vi "Close-file.vi"(8 "error in (no error)":errorcluster, 11 "SettingsFile in":refnum<class "SettingsFile.lvclass">) -> (0 "error out":errorcluster, 3 "SettingsFile out":refnum<class "SettingsFile.lvclass">)   [LabVIEW 2013, in "SettingsFile.lvlib" / "SettingsFile.lvclass"]
uses:
  SettingsFile.lvclass
  SettingsFile.lvclass/SettingsFile.ctl
  Errors.ctl
  <vilib>/Utility/config.llb/Config Data RefNum.ctl
  <vilib>/Utility/config.llb/NI_LVConfig.lvlib
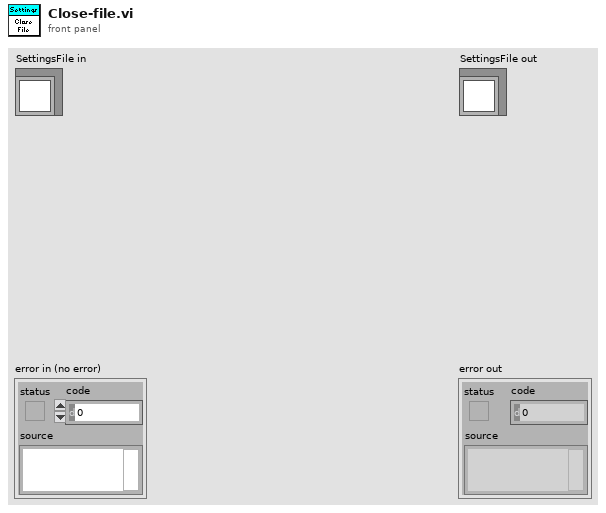
[diagram p1: front panel]
types:
  T1 = typedef "SettingsFile.lvlib/SettingsFile.lvclass/Errors.ctl" = enum16{"Not implemented", "Command not recognized", "Invalid input", "No connection", "Timeout", "Invalid file type", "No file access"}
  T2 = typedef "NI_LVConfig.lvlib/Config Data RefNum.ctl" = refnum<k1>
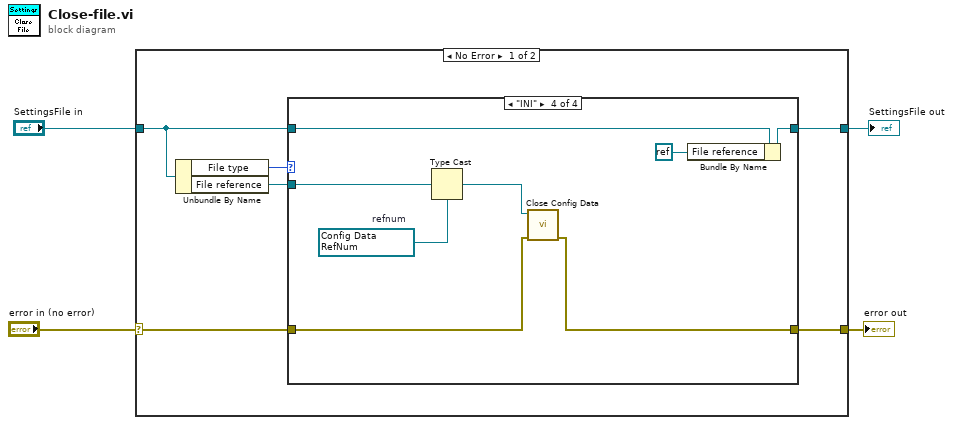
[diagram p0: block diagram]
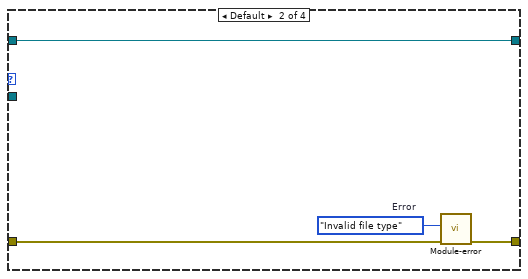
[diagram p3: hidden frame]
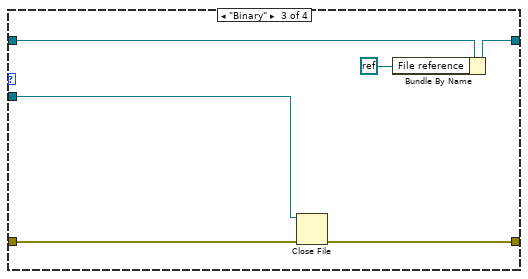
[diagram p4: hidden frame]
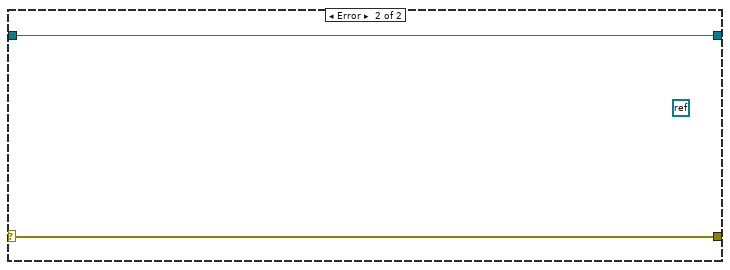
[diagram p5: hidden frame]
diagram:
  n1 = case shown="No Error" "error in (no error)" {
    selector: "error in (no error)" -> [w10 w32]
    tunnel: [w9 w32] -> w3
    tunnel: [w8 w31] -> w1
    tunnel: "SettingsFile in" -> [w7 w31]
    frame No Error {
      n2 = Unbundle By Name(w7) -> ("File type"=w6:enum16{"XML", "INI", "Binary"}, "File reference"=w5:refnum<file>)
      n3 = case shown="\"INI\"" w6 {
        tunnel: w7 -> [w12 w16 w22 w30]
        tunnel: w10 -> [w11 w14 w20 w27]
        tunnel: [w11 w15 w19 w26] -> w9
        tunnel: [w12 w16 w21 w29] -> w8
        tunnel: w5 -> [_ _ w18 w28]
        frame "XML" {
        }
        frame Default {
          w13 = Errors."Invalid file type"  # Error
          n4 = call "Module-error.vi"("error in (no error)"=w14, "Error"=w13) -> ("error out"=w15:errorcluster)  [unwired: 9 in]
        }
        frame "Binary" {
          n5 = Close File(refnum=w18, error in=w20) -> (error out=w19:errorcluster)  [unwired: 1 out]
          n6 = Bundle By Name(cluster=w22, "File reference"=refnum<k0> refnum) -> (w21:refnum<class "SettingsFile.lvclass">)
        }
        frame "INI" {
          w25 = T2 refnum items=["config data"]  # refnum
          n7 = Type Cast(type=w25, x=w28) -> (*(type *) &x=w24:T2)
          n8 = call <vilib>:"Close Config Data.vi"("error in (no error)"=w27, "refnum"=w24) -> ("error out"=w26:errorcluster)  [unwired: 8 in, 1 out]
          n9 = Bundle By Name(cluster=w30, "File reference"=refnum<k0> refnum) -> (w29:refnum<class "SettingsFile.lvclass">)
        }
      }
    }
    frame Error {
      (unwired) refnum<k0> refnum
    }
  }
  "error out" <- w3
  "SettingsFile out" <- w1
